vi "sendAckNoAckToClient.vi"(8 "error in (no error)":errorcluster, 9 "ackIterations":i32, 10 "tcpPacket":T1, 11 "tcpServerCmd in":refnum<class "TcpServerCmd.lvclass">) -> (0 "error out":errorcluster, 3 "tcpServerCmd out":refnum<class "TcpServerCmd.lvclass">)   [LabVIEW 2018, in "TcpServerCmd.lvclass"]
doc: "Send the ack to the TCP Client for the last command received, and if there are lost commands, it sends noAck for them."
uses:
  TcpServerCmd.lvclass
  TcpServerBase/typedef/tcpPacketTypeDef.ctl
  TcpServerBase/TcpServerBase.lvclass
panel:
  out "tcpPacket":T1
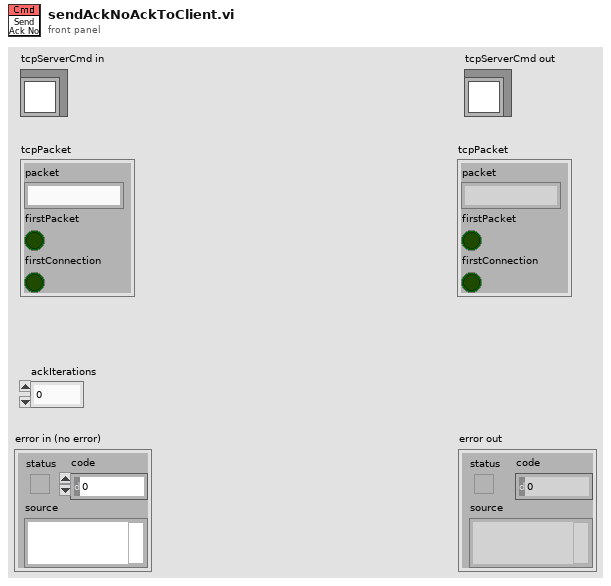
[diagram p1: front panel]
types:
  T1 = typedef "TcpServerBase.lvclass/tcpPacketTypeDef.ctl" = cluster{"packet":string, "firstPacket":bool, "firstConnection":bool}
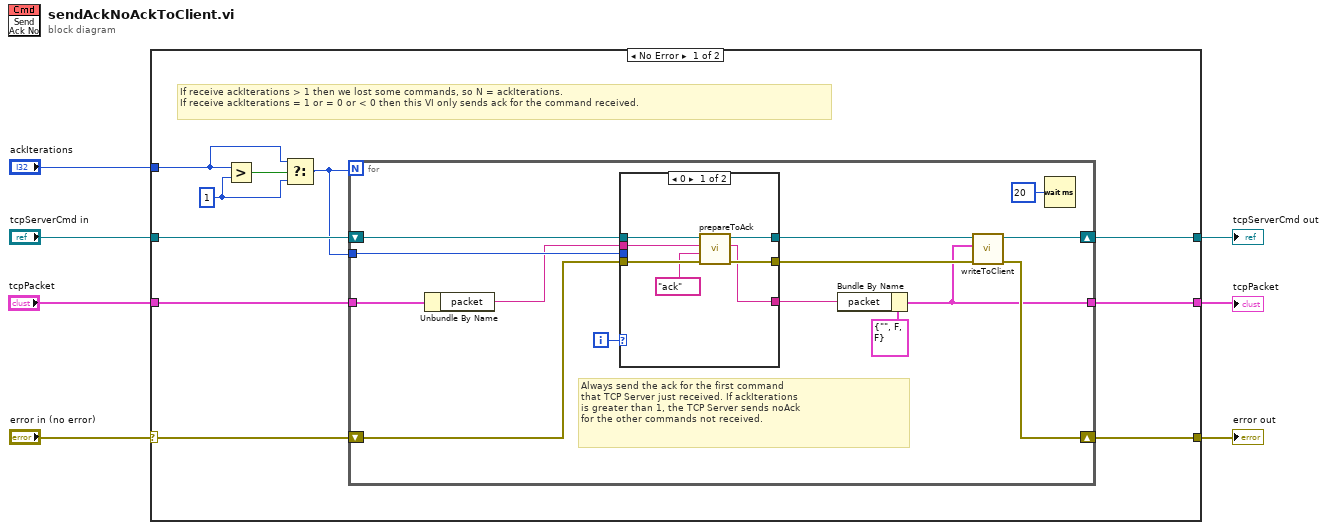
[diagram p0: block diagram]
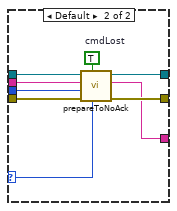
[diagram p2: hidden frame]
diagram:
  n1 = case shown="No Error" "error in (no error)" {
    selector: "error in (no error)" -> [w17 w48]
    tunnel: [w16 w48] -> w6
    tunnel: "tcpServerCmd in" -> [w15 w50]
    tunnel: [w14 w50] -> w4
    tunnel: "tcpPacket" -> [w13 w49]
    tunnel: [w12 w49] -> w1
    tunnel: "ackIterations" -> [w10 _]
    frame No Error {
      w9 = 1 ("y")
      # "If receive ackIterations > 1 then we lost some commands, so N = ackIterations.\nIf receive ackIterations = 1 or = 0 or < 0 then this VI only sends ack for the command received."
      n2 = Greater?(x=w10, y=w9) -> (0:w11:bool)
      n3 = Select(t=w10, s=w11, f=w9) -> (s? t:f=w8:i32)
      n4 = for {
        N: w8 -> [_]
        tunnel: w13 -> [w27]
        tunnel: w8 -> [w26]
        shift-right: [w30] -> w16
        shift-left: w17 -> [w31]
        shift-right: [w28] -> w14
        shift-left: w15 -> [w29]
        tunnel: [w19] -> w12
        i -> [w20]
        # "Always send the ack for the first command\nthat TCP Server just received. If ackIterations\nis greater than 1, the TCP Server sends noAck \nfor the other commands not received."
        n5 = Unbundle By Name(w27) -> ("packet"=w23:string)
        n6 = case shown="0" w20 {
          selector: w20 -> [_ w40]
          tunnel: w31 -> [w36 w47]
          tunnel: w29 -> [w38 w46]
          tunnel: w26 -> [_ w45]
          tunnel: [w37 w44] -> w25
          tunnel: [w35 w43] -> w24
          tunnel: w23 -> [w34 w42]
          tunnel: [w33 w41] -> w22
          frame 0 {
            n7 = call "prepareToAck.vi"("error in (no error)"=w36, "cmdStatus"="ack", "cmd"=w34, "tcpServerCmd in"=w38) -> ("error out"=w35:errorcluster, "JSON string"=w33:string, "tcpServerCmd out"=w37:refnum<class "TcpServerCmd.lvclass">)  [unwired: 5 in]
          }
          frame Default {
            w39 = TRUE  # cmdLost
            n8 = call "prepareToNoAck.vi"("iteration"=w40, "cmdLost"=w39, "error in (no error)"=w47, "lostCmdId"=w45, "cmd"=w42, "tcpServerCmd in"=w46) -> ("error out"=w43:errorcluster, "JSON string"=w41:string, "tcpServerCmd out"=w44:refnum<class "TcpServerCmd.lvclass">)  [unwired: 3 in]
          }
        }
        n9 = Bundle By Name(cluster=T1 {"packet"="", "firstPacket"=FALSE, "firstConnection"=FALSE} ("tcpPacket"), "packet"=w22) -> (w19:T1)
        n10 = call "writeToClient.vi"("error in (no error)"=w24, "tcpPacket"=w19, "tcpServerCmd in"=w25) -> ("error out"=w30:errorcluster, "tcpServerCmd out"=w28:refnum<class "TcpServerCmd.lvclass">)  [unwired: 7 in]
        n11 = Wait (ms)(milliseconds to wait=u32 20) -> ()  [unwired: 1 out]
      }
    }
    frame Error {
    }
  }
  "error out" <- w6
  "tcpServerCmd out" <- w4
  "tcpPacket" <- w1
